vi "Write Pin.vi"(0 "Serial Device in":refnum<class "Serial Device.lvclass">, 5 "VISA resource name":refnum<visa-resource-name>, 7 "Pin":u16, 9 "Port 3":u16, 11 "error in (no error)":errorcluster, 12 "Set Pin":bool) -> (4 "Serial Device out":refnum<class "Serial Device.lvclass">, 6 "VISA resource name 2":refnum<visa-resource-name>, 15 "error out":errorcluster)   [LabVIEW 2020, in "Serial Device.lvclass"]
uses:
  Serial Device.lvclass
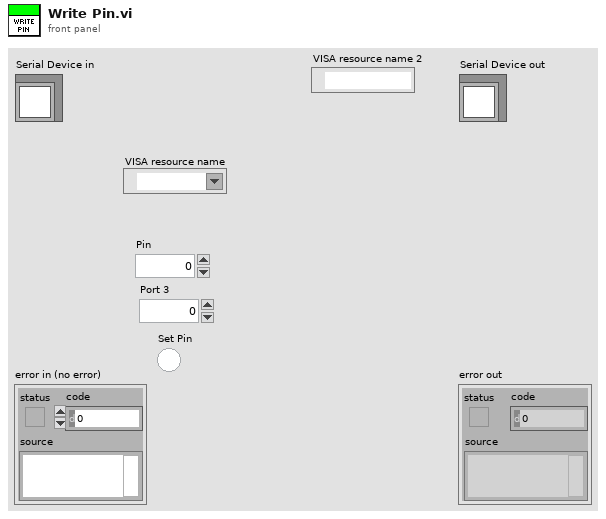
[diagram p1: front panel]
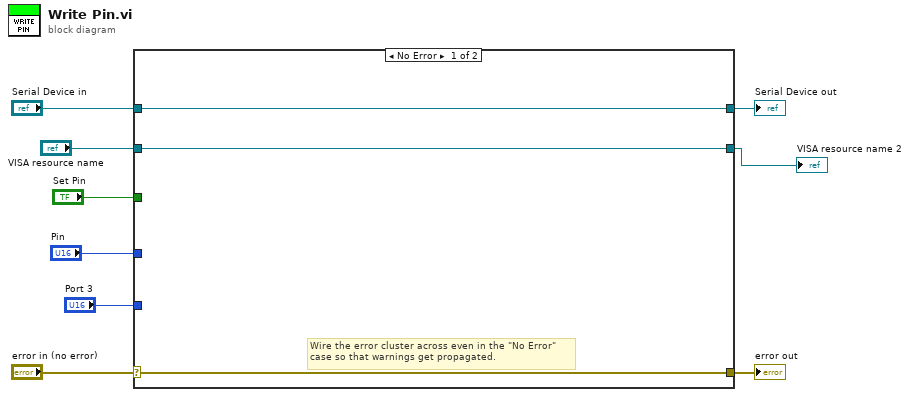
[diagram p0: block diagram]
diagram:
  n1 = case shown="No Error" "error in (no error)" {
    selector: "error in (no error)" -> [w11 w15]
    tunnel: [w11 w15] -> w8
    tunnel: [w12 w14] -> w6
    tunnel: "Serial Device in" -> [w12 w14]
    tunnel: "Pin" -> [_ _]
    tunnel: "Set Pin" -> [_ _]
    tunnel: "Port 3" -> [_ _]
    tunnel: "VISA resource name" -> [w10 w13]
    tunnel: [w10 w13] -> w1
    frame No Error {
      # "Wire the error cluster across even in the \"No Error\"\ncase so that warnings get propagated."
    }
    frame Error {
    }
  }
  "error out" <- w8
  "Serial Device out" <- w6
  "VISA resource name 2" <- w1
